vi "Broadcast Flow Settings.vi"(8 "error in (no error)":errorcluster, 10 "Message Queues":T6, 11 "Flow Module Config":T1={"GUID"="", "Drop Coords"={"Horizontal"=0, "Vertical"=0}, "Process Name"="", "Queue Name"="", "Settings"={"Cycle Period"=500.0, "Flow Meter Type"="", "Bronkhorst M13 Settings"={"VISA resource name"="", "Simulated?"=FALSE, "Smoothing Steps"=1}, "Bronkhorst M14 Settings"={"VISA resource name"="", "Simulated?"=FALSE, "Smoothing Steps"=1}}, "Load Count"=0} {"Settings"."Bronkhorst M14 Settings"."Smoothing Steps" min=1 step=1; "Settings"."Bronkhorst M13 Settings"."Smoothing Steps" min=1 step=1}) -> (0 "error out":errorcluster)   [LabVIEW 2018, in "Flow Module.lvlib"]
uses:
  Flow Module.lvlib
  Flow Message Queues.ctl
  support/Message Queue/Message Cluster.ctl
  Controls/Flow Module Config Cluster.ctl
  <vilib>/Utility/miscctls.llb/LVPoint32TypeDef.ctl
  Controls/Flow Module Settings Cluster.ctl
  Bronkhorst M13 Flow Meter/Settings Cluster.ctl
  Bronkhorst M14 Flow Meter/Settings Cluster.ctl
  support/Message Queue/Enqueue Message (Single).vi
  support/Message Queue/Message Queue.lvlib
  Bronkhorst M13 Flow Meter/Bronkhorst M13 Flow Meter.lvlib
  Bronkhorst M14 Flow Meter/Bronkhorst M14 Flow Meter.lvlib
panel:
  # "Flow Meter Settings"
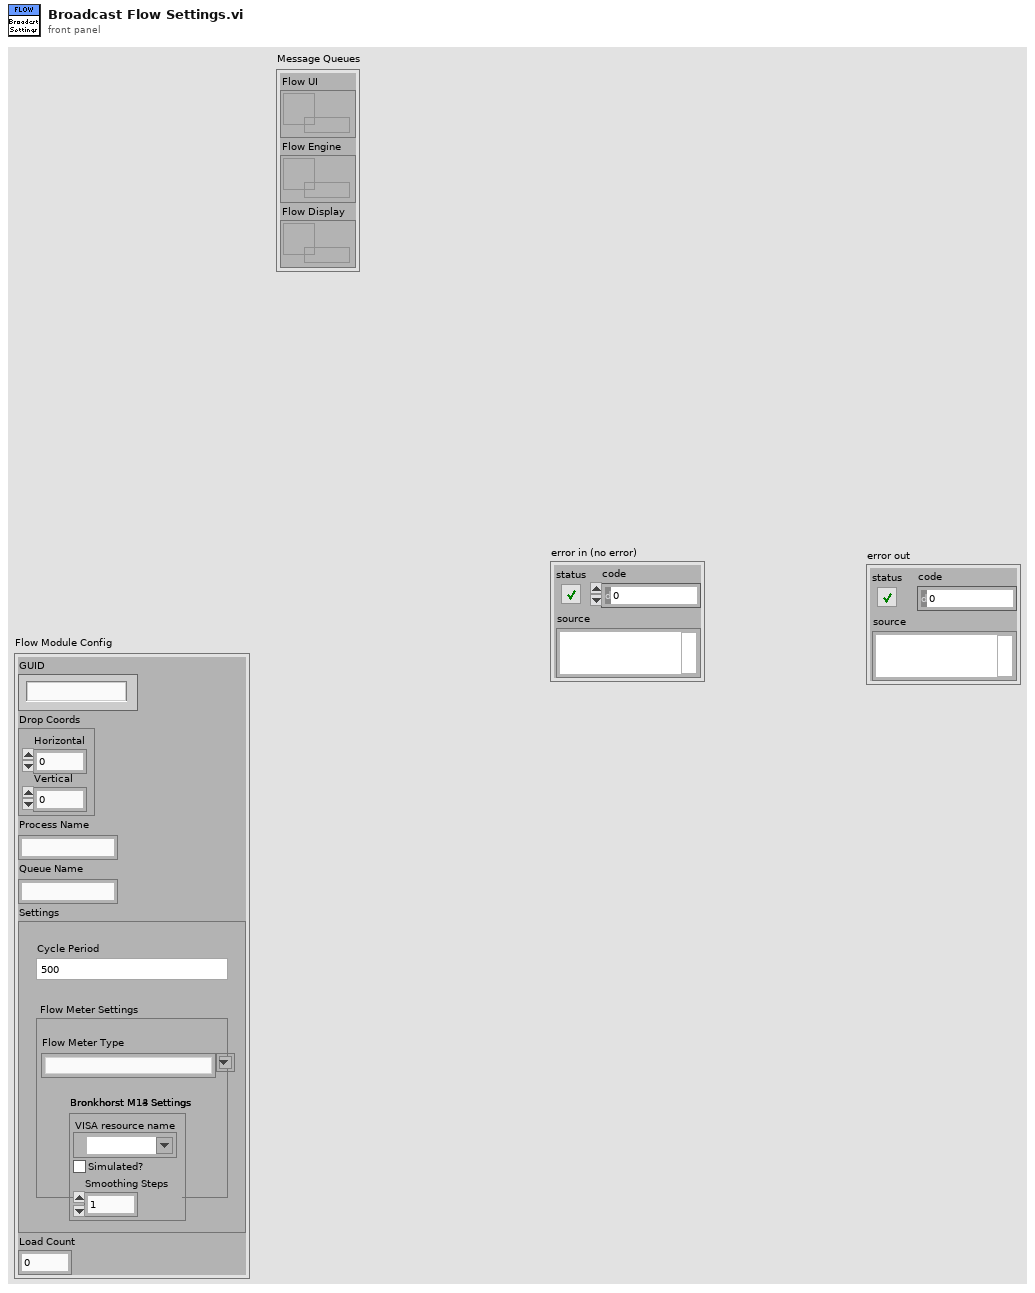
[diagram p1: front panel]
types:
  T1 = typedef "Flow Module.lvlib/Flow Module Config Cluster.ctl" = cluster{"GUID":string, "Drop Coords":T2, "Process Name":string, "Queue Name":string, "Settings":T3, "Load Count":i32}
  T2 = typedef "LVPoint32TypeDef.ctl" = cluster{"Horizontal":i32, "Vertical":i32}
  T3 = typedef "Flow Module.lvlib/Flow Module Settings Cluster.ctl" = cluster{"Cycle Period":dbl, "Flow Meter Type":string, "Bronkhorst M13 Settings":T4, "Bronkhorst M14 Settings":T5}
  T4 = typedef "Bronkhorst M13 Flow Meter.lvlib/Settings Cluster.ctl" = cluster{"VISA resource name":refnum<visa-resource-name>, "Simulated?":bool, "Smoothing Steps":i32}
  T5 = typedef "Bronkhorst M14 Flow Meter.lvlib/Settings Cluster.ctl" = cluster{"VISA resource name":refnum<visa-resource-name>, "Simulated?":bool, "Smoothing Steps":i32}
  T6 = typedef "Flow Module.lvlib/Flow Message Queues.ctl" = cluster{"Flow UI":refnum<queue>, "Flow Engine":refnum<queue>, "Flow Display":refnum<queue>}
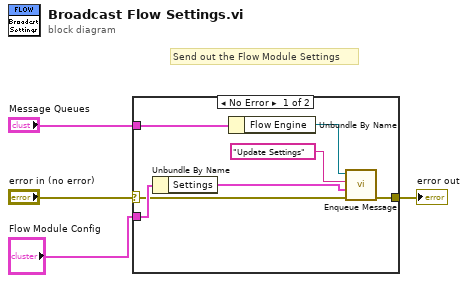
[diagram p0: block diagram]
diagram:
  # "Send out the Flow Module Settings"
  n1 = case shown="No Error" "error in (no error)" {
    selector: "error in (no error)" -> [w6 w12]
    tunnel: [w5 w12] -> w2
    tunnel: "Flow Module Config" -> [w11 _]
    tunnel: "Message Queues" -> [w10 _]
    frame No Error {
      n2 = Unbundle By Name(w11) -> ("Settings"=w8:T3)
      n3 = Unbundle By Name(w10) -> ("Flow Engine"=w9:refnum<queue>)
      n4 = call-poly "Enqueue Message.vi"("error in (no error)"=w6, "Message Data"=w8, "Message"="Update Settings", "Message Queue"=w9) -> ("error out"=w5:errorcluster)  [unwired: 6 in, 1 out]
    }
    frame Error {
    }
  }
  "error out" <- w2
